vi "Stack.vi"   [LabVIEW 2016, in "Moving Motor.lvrbt"]
uses:
  Moving Motor.lvrbt
  <vilib>/NXT/Hardware/Plugins/Tetrix 180 deg Servo/Tetrix180ServoAddress.ctl
  <vilib>/NXT/Hardware/Plugins/Tetrix DC Motor/TetrixDCMotorAddress.ctl
  <vilib>/NXT/NXTIO Xnodes/NXTIONodeSubVIs/TETRIX IO Move Servos.vi
  <vilib>/NXT/NXTIO Xnodes/NXTIONodeSubVIs/TETRIX IO Move DC Motors.vi
  <vilib>/NXT/NXTIO Xnodes/NXTIONodeSubVIs/TETRIX IO Stop DC Motors.vi
  <vilib>/NXT/Subs/LVHSConnector.ctl
  <vilib>/NXT/NXTIO Xnodes/AddressXNode/NXTIOAddress.xnode
  <vilib>/NXT/NXTIO Xnodes/NXTIOXNode/NXTIO.xnode
  <vilib>/NXT/LegoClasses/BrickReference/BrickReference.lvclass
types:
  T1 = typedef "Tetrix180ServoAddress.ctl" = i32
  T2 = cluster{"Tetrix180Servo":T1, "Tetrix180Servo":T1}
  T3 = typedef "LVHSConnector.ctl" = refnum<class "BrickReference.lvclass">
  T4 = typedef "TetrixDCMotorAddress.ctl" = i32
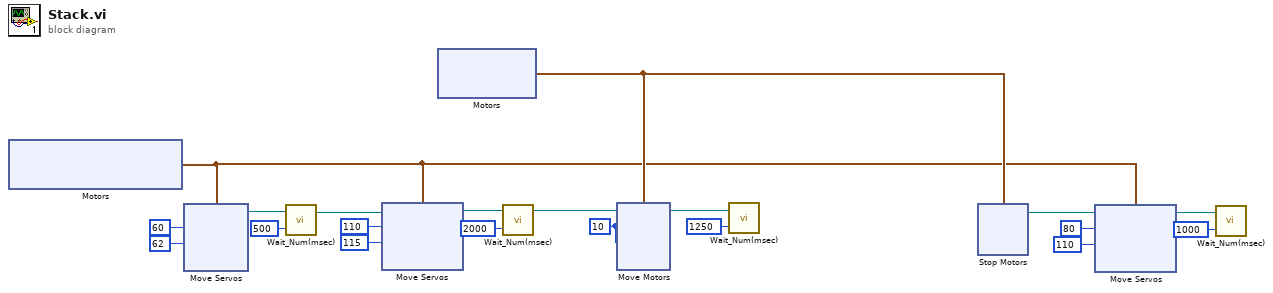
[diagram p0: block diagram]
diagram:
  w10 = i8 10 ("Power/Speed 1")
  n1 = xnode "Motors"() -> ("Motor"=w5:T2)
  n2 = xnode "Move Servos"("Position 2"=u8 62, "Position 1"=u8 60, "Motors"=w5) -> ("NXT/EV3"=w18:T3)  [unwired: 1 in]
  n3 = call <vilib>:"Wait_Num(msec).vi"("Time (100 msec)"=u32 500, "NXT/EV3"=w18) -> ("NXT/EV3"=w15:T3)  [unwired: 2 in]
  n4 = xnode "Move Servos"("Position 2"=u8 115, "Position 1"=u8 110, "Motors"=w5, "NXT/EV3"=w15) -> ("NXT/EV3"=w12:T3)
  n5 = xnode "Motors"() -> ("Motor"=w7:cluster{"TetrixDCMotor":T4, "TetrixDCMotor":T4})
  n6 = call <vilib>:"Wait_Num(msec).vi"("Time (100 msec)"=u32 2000, "NXT/EV3"=w12) -> ("NXT/EV3"=w11:T3)  [unwired: 2 in]
  n7 = xnode "Move Motors"("Power/Speed 2"=w10, "Power/Speed 1"=w10, "Motors"=w7, "NXT/EV3"=w11) -> ("NXT/EV3"=w8:T3)
  n8 = call <vilib>:"Wait_Num(msec).vi"("Time (100 msec)"=u32 1250, "NXT/EV3"=w8) -> ()  [unwired: 2 in, 1 out]
  n9 = xnode "Stop Motors"("Motors"=w7) -> ("NXT/EV3"=w3:T3)  [unwired: 1 in]
  n10 = xnode "Move Servos"("Position 2"=u8 110, "Position 1"=u8 80, "Motors"=w5, "NXT/EV3"=w3) -> ("NXT/EV3"=w1:T3)
  n11 = call <vilib>:"Wait_Num(msec).vi"("Time (100 msec)"=u32 1000, "NXT/EV3"=w1) -> ()  [unwired: 2 in, 1 out]
